vi "Mouse toggle X-Y for calibration.vi"(8 "error in (no error) 3":errorcluster) -> ()   [LabVIEW 2011]
panel:
  in  "Set diode pos":bool
  in  "Go to negative limit":bool
  out "Y Pos":string
  out "X Pos":string
  out "Enabled?":bool
  in  "Enable Motors":bool
  in  "Y -ve":bool
  in  "Y +ve":bool
  in  "X -ve":bool
  in  "X +ve":bool
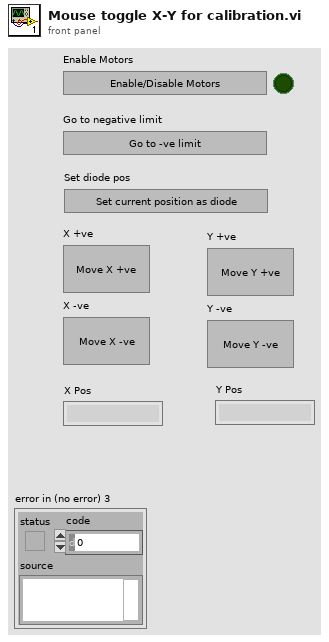
[diagram p1: front panel]
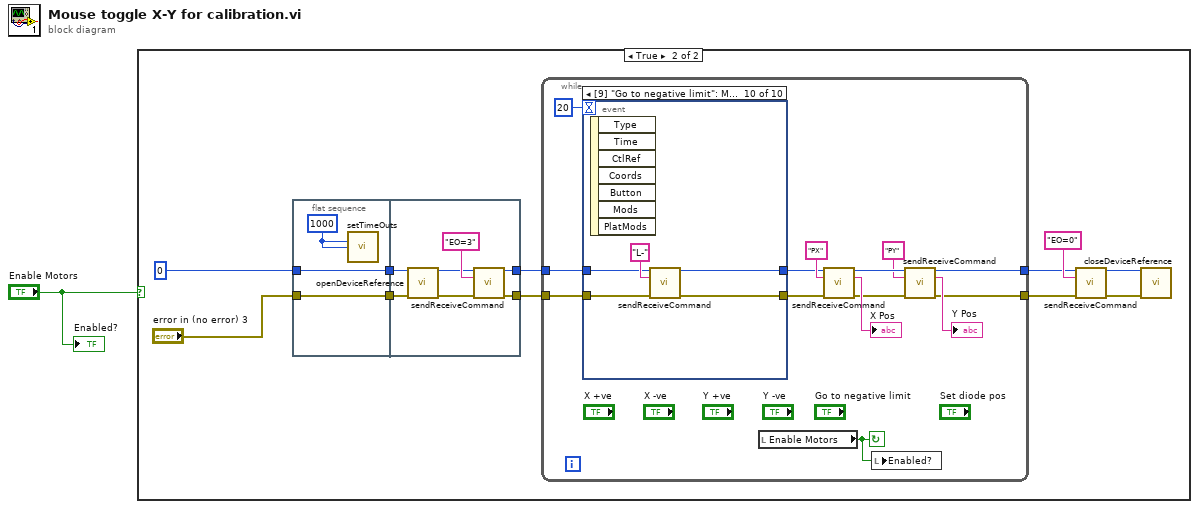
[diagram p0: block diagram]
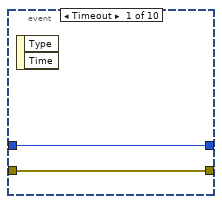
[diagram p3: hidden frame]
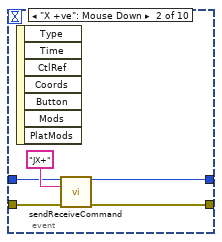
[diagram p4: hidden frame]
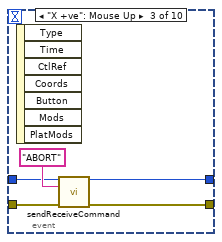
[diagram p5: hidden frame]
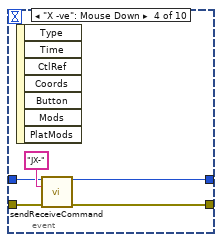
[diagram p6: hidden frame]
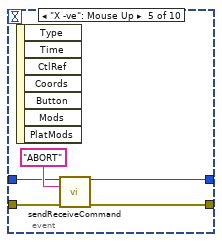
[diagram p7: hidden frame]
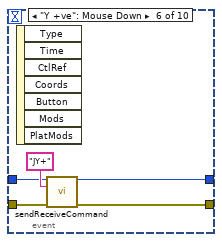
[diagram p8: hidden frame]
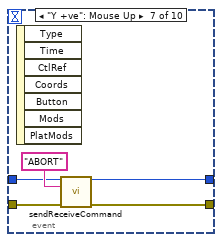
[diagram p9: hidden frame]
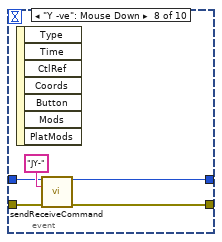
[diagram p10: hidden frame]
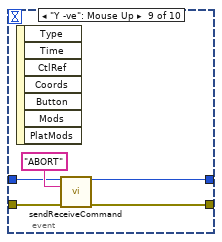
[diagram p11: hidden frame]
diagram:
  n1 = case shown="True" "Enable Motors" {
    frame False {
    }
    frame True {
      n2 = flat-sequence {
        tunnel: 0 -> [w14]
        tunnel: [w14] -> w12
        tunnel: "error in (no error) 3" -> [w13]
        tunnel: [w13] -> w11
        tunnel: w12 -> [w22]
        tunnel: w11 -> [w21]
        tunnel: [w19] -> w8
        tunnel: [w18] -> w7
        frame #0 {
          w15 = 1000 ("read_timeout")
          n3 = call "setTimeOuts.vi"("read_timeout (ms)"=w15, "write_timeout (ms)"=w15) -> ()  [unwired: 13 in, 1 out]
        }
        frame #1 {
          n4 = call "openDeviceReference.vi"("deviceIndex"=w22, "error in (no error)"=w21) -> ("reference"=w17:i32, "error out"=w16:errorcluster)  [unwired: 12 in]
          n5 = call "sendReceiveCommand.vi"("reference (in)"=w17, "write_string"="EO=3" ("raw_cmd 2"), "error in (no error)"=w16) -> ("reference (out)"=w19:i32, "error out"=w18:errorcluster)  [unwired: 10 in, 1 out]
        }
      }
      n6 = while {
        tunnel: w8 -> [w36]
        tunnel: w7 -> [w35]
        tunnel: [w24] -> w3
        tunnel: [w23] -> w2
        stop <- w33 continue-if-true
        n7 = event shown="[9] \"Go to negative limit\": Mouse Down" {
          selector: _ -> [_ _ _ _ _ _ _ _ _ _]
          dyn-events: _ -> [_ _ _ _ _ _ _ _ _ _]
          timeout: 20 -> [_ _ _ _ _ _ _ _ _ _]
          tunnel: w36 -> [w38 w42 w47 w52 w57 w62 w67 w72 w77 w82]
          tunnel: w35 -> [w37 w41 w46 w51 w56 w61 w66 w71 w76 w81]
          tunnel: [w38 w40 w45 w50 w55 w60 w65 w70 w75 w80] -> w30
          tunnel: [w37 w39 w44 w49 w54 w59 w64 w69 w74 w79] -> w29
          event Timeout {
            n8 = event-data() -> ()  [unwired: 1 in, 2 out]
          }
          event "X +ve": Mouse Down {
            n9 = event-data() -> ()  [unwired: 1 in, 7 out]
            n10 = call "sendReceiveCommand.vi"("reference (in)"=w42, "write_string"="JX+" ("raw_cmd"), "error in (no error)"=w41) -> ("reference (out)"=w40:i32, "error out"=w39:errorcluster)  [unwired: 10 in, 1 out]
          }
          event "X +ve": Mouse Up {
            n11 = event-data() -> ()  [unwired: 1 in, 7 out]
            n12 = call "sendReceiveCommand.vi"("reference (in)"=w47, "write_string"="ABORT" ("raw_cmd"), "error in (no error)"=w46) -> ("reference (out)"=w45:i32, "error out"=w44:errorcluster)  [unwired: 10 in, 1 out]
          }
          event "X -ve": Mouse Down {
            n13 = event-data() -> ()  [unwired: 1 in, 7 out]
            n14 = call "sendReceiveCommand.vi"("reference (in)"=w52, "write_string"="JX-" ("raw_cmd"), "error in (no error)"=w51) -> ("reference (out)"=w50:i32, "error out"=w49:errorcluster)  [unwired: 10 in, 1 out]
          }
          event "X -ve": Mouse Up {
            n15 = event-data() -> ()  [unwired: 1 in, 7 out]
            n16 = call "sendReceiveCommand.vi"("reference (in)"=w57, "write_string"="ABORT" ("raw_cmd"), "error in (no error)"=w56) -> ("reference (out)"=w55:i32, "error out"=w54:errorcluster)  [unwired: 10 in, 1 out]
          }
          event "Y +ve": Mouse Down {
            n17 = event-data() -> ()  [unwired: 1 in, 7 out]
            n18 = call "sendReceiveCommand.vi"("reference (in)"=w62, "write_string"="JY+" ("raw_cmd"), "error in (no error)"=w61) -> ("reference (out)"=w60:i32, "error out"=w59:errorcluster)  [unwired: 10 in, 1 out]
          }
          event "Y +ve": Mouse Up {
            n19 = event-data() -> ()  [unwired: 1 in, 7 out]
            n20 = call "sendReceiveCommand.vi"("reference (in)"=w67, "write_string"="ABORT" ("raw_cmd"), "error in (no error)"=w66) -> ("reference (out)"=w65:i32, "error out"=w64:errorcluster)  [unwired: 10 in, 1 out]
          }
          event "Y -ve": Mouse Down {
            n21 = event-data() -> ()  [unwired: 1 in, 7 out]
            n22 = call "sendReceiveCommand.vi"("reference (in)"=w72, "write_string"="JY-" ("raw_cmd"), "error in (no error)"=w71) -> ("reference (out)"=w70:i32, "error out"=w69:errorcluster)  [unwired: 10 in, 1 out]
          }
          event "Y -ve": Mouse Up {
            n23 = event-data() -> ()  [unwired: 1 in, 7 out]
            n24 = call "sendReceiveCommand.vi"("reference (in)"=w77, "write_string"="ABORT" ("raw_cmd"), "error in (no error)"=w76) -> ("reference (out)"=w75:i32, "error out"=w74:errorcluster)  [unwired: 10 in, 1 out]
          }
          event "Go to negative limit": Mouse Down {
            n25 = event-data() -> ()  [unwired: 1 in, 7 out]
            n26 = call "sendReceiveCommand.vi"("reference (in)"=w82, "write_string"="L-" ("raw_cmd"), "error in (no error)"=w81) -> ("reference (out)"=w80:i32, "error out"=w79:errorcluster)  [unwired: 10 in, 1 out]
          }
        }
        n27 = local read "Enable Motors"() -> (w33:bool)
        n28 = call "sendReceiveCommand.vi"("reference (in)"=w30, "write_string"="PX" ("raw_cmd"), "error in (no error)"=w29) -> ("reference (out)"=w27:i32, "read_string"=→"X Pos":string, "error out"=w26:errorcluster)  [unwired: 10 in]
        n29 = local write "Enabled?"(w33) -> ()
        n30 = call "sendReceiveCommand.vi"("reference (in)"=w27, "write_string"="PY" ("raw_cmd"), "error in (no error)"=w26) -> ("reference (out)"=w24:i32, "read_string"=→"Y Pos":string, "error out"=w23:errorcluster)  [unwired: 10 in]
      }
      n31 = call "sendReceiveCommand.vi"("reference (in)"=w3, "write_string"="EO=0" ("raw_cmd 2"), "error in (no error)"=w2) -> ("reference (out)"=w5:i32, "error out"=w4:errorcluster)  [unwired: 10 in, 1 out]
      n32 = call "closeDeviceReference.vi"("reference"=w5, "error in (no error)"=w4) -> ()  [unwired: 13 in, 1 out]
    }
  }
  "Enabled?" <- "Enable Motors"
